vi "gantry path main.vi"() -> ()   [LabVIEW 2016]
uses:
  Classes/Controller/Motion/A3200 Folder/A3200.lvclass
  D:/Gantry_General/Classes/Controller/Motion/Motion Folder/Motion.lvclass
  Classes/Controller/Dispenser/Ultimus V2 Folder/Ultimus V2.lvclass
  Classes/Controller/I-O/NI-DAQ Folder/NI-DAQ.lvclass
  Classes/Controller/Motion/Motion Folder/Motion.lvclass
  Classes/Controller/I-O/I-O Folder/I-O.lvclass
  Classes/Controller/Dispenser/Dispenser Folder/Dispenser.lvclass
  <vilib>/Utility/file.llb/Read Delimited Spreadsheet (DBL).vi
  <vilib>/Utility/file.llb/Write Delimited Spreadsheet (DBL).vi
panel:
  out "run XYZTheta Out":dbl[](array[numeric])
  in  "string":string
  out "new path":path=path "D:/Gantry_General/Main/ms_kao/gantry path/path data/20211104-170200.046.txt"
  out "array w/ subset deleted":dbl[](array[numeric])=[1038.895, 600.353]
  out "deleted portion":dbl[](array[numeric])=[51.418, -0.0]
  out "subarray":dbl[](array[numeric])=[-0.016895, 380.054641, 0.0, -0.0]
  out "all rows":dbl[][](array[numeric])=[[1e-06, -9e-06, 0.0, 0.0], [380.023807, -5.6e-05, 1e-06, -0.0], [380.005908, 380.030345, 0.0, 1e-06], [-0.016895, 380.054641, 0.0, -0.0]]
  out "size(s)":i32[](array[numeric])=[4, 4]
  in  "cul data":bool
  in  "Tab Control":enum32{"controller", "path", "motion"}(tab)=enum."motion"
  in  "controller":T1
  in  "save data off/on":bool=TRUE
  in  "test / run 2":bool
  out "run":bool
  out "XYZU":dbl[](array[numeric])=[388.99999394968614, 389.00001276830227, 35.37117897777896, -9.350854999021411e-05]
  in  "joystick":bool
  out "Axis 2":dbl[](array[numeric])=[388.99999394968614, 389.00001276830227, 35.37117897777896, -9.350854999021411e-05]
  in  "get Axis":bool
  in  "get origin":bool
  in  "test / run":bool=TRUE
  in  "joystick off/on":bool=TRUE
  in  "XY / XYZXU":bool
  in  "Read old path":path=path "D:/Gantry_General/Main/ms_kao/gantry path/path data/20220615/calibration meterial20220111_.txt"
  in  "go path":bool
  in  "milliseconds to wait":u32=500
  out "Origin":dbl[](array[numeric])=[388.999994, 389.000013, 35.371179, -9.4e-05]
  out "file or folder exists?":bool=TRUE
  in  "add new path":bool
  in  "XY go2":bool
  in  "XYZU Position":dbl[](array[numeric])=[500.0, 500.0, 0.0]
  in  "Z Speed":dbl=40.0
  in  "XY go1":bool
  in  "XYZU go":bool
  in  "Z go":bool
  in  "XY Speed":dbl=100.0
  in  "Z Position":dbl format="%#_13g"
  in  "XY Position 1":dbl[](array[numeric])=[687.973, 195.062]
  in  "XY Position 2":dbl[](array[numeric])=[687.973, 252.062]
  in  "stop":bool
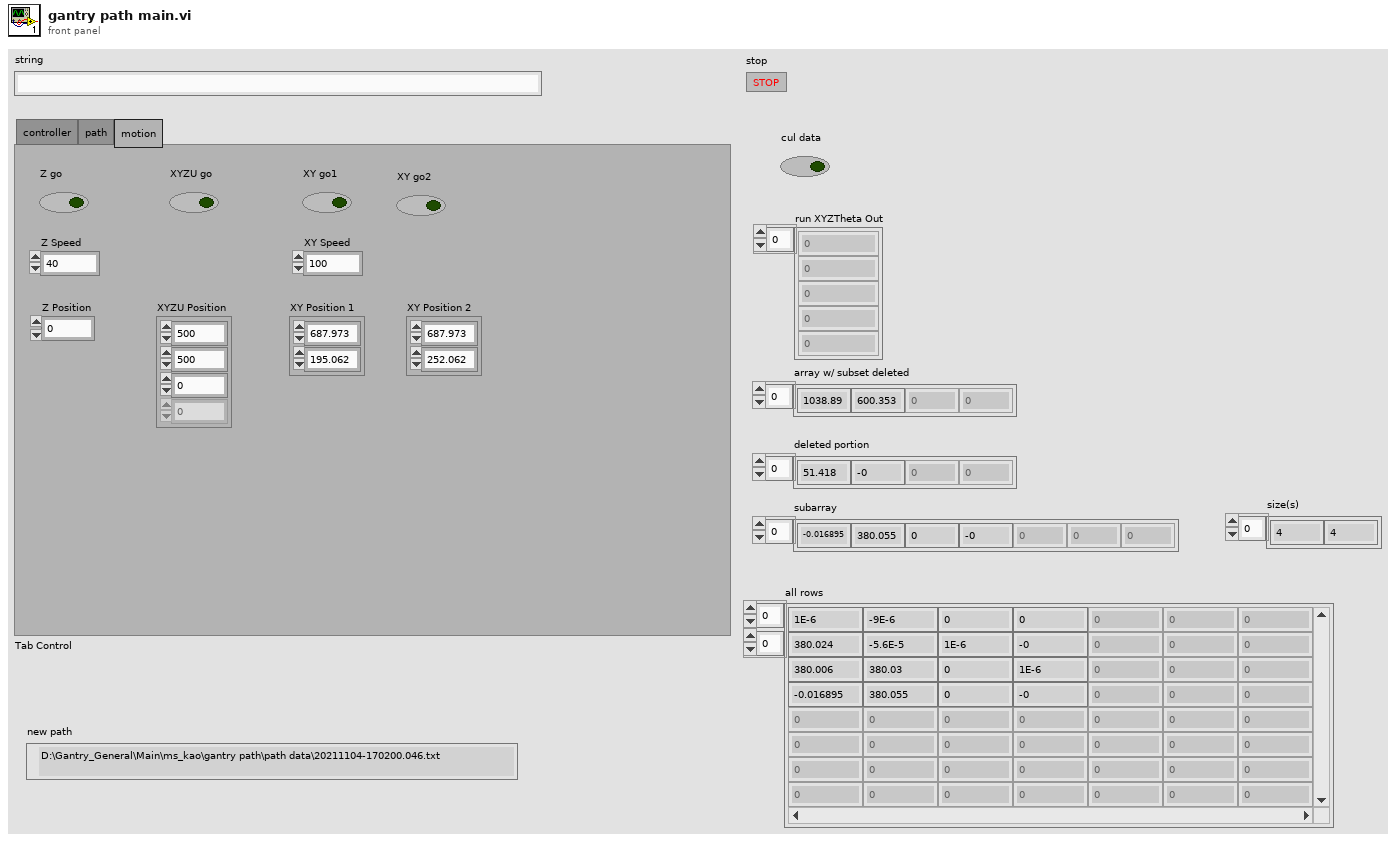
[diagram p1: front panel]
types:
  T1 = cluster{"A3200.lvclass":refnum<class "A3200.lvclass">, "Ultimus V2.lvclass":refnum<class "Ultimus V2.lvclass">, "NI-DAQ.lvclass":refnum<class "NI-DAQ.lvclass">, "Motion.lvclass":refnum<class "Motion.lvclass">, "I-O.lvclass":refnum<class "I-O.lvclass">, "Dispenser.lvclass":refnum<class "Dispenser.lvclass">}
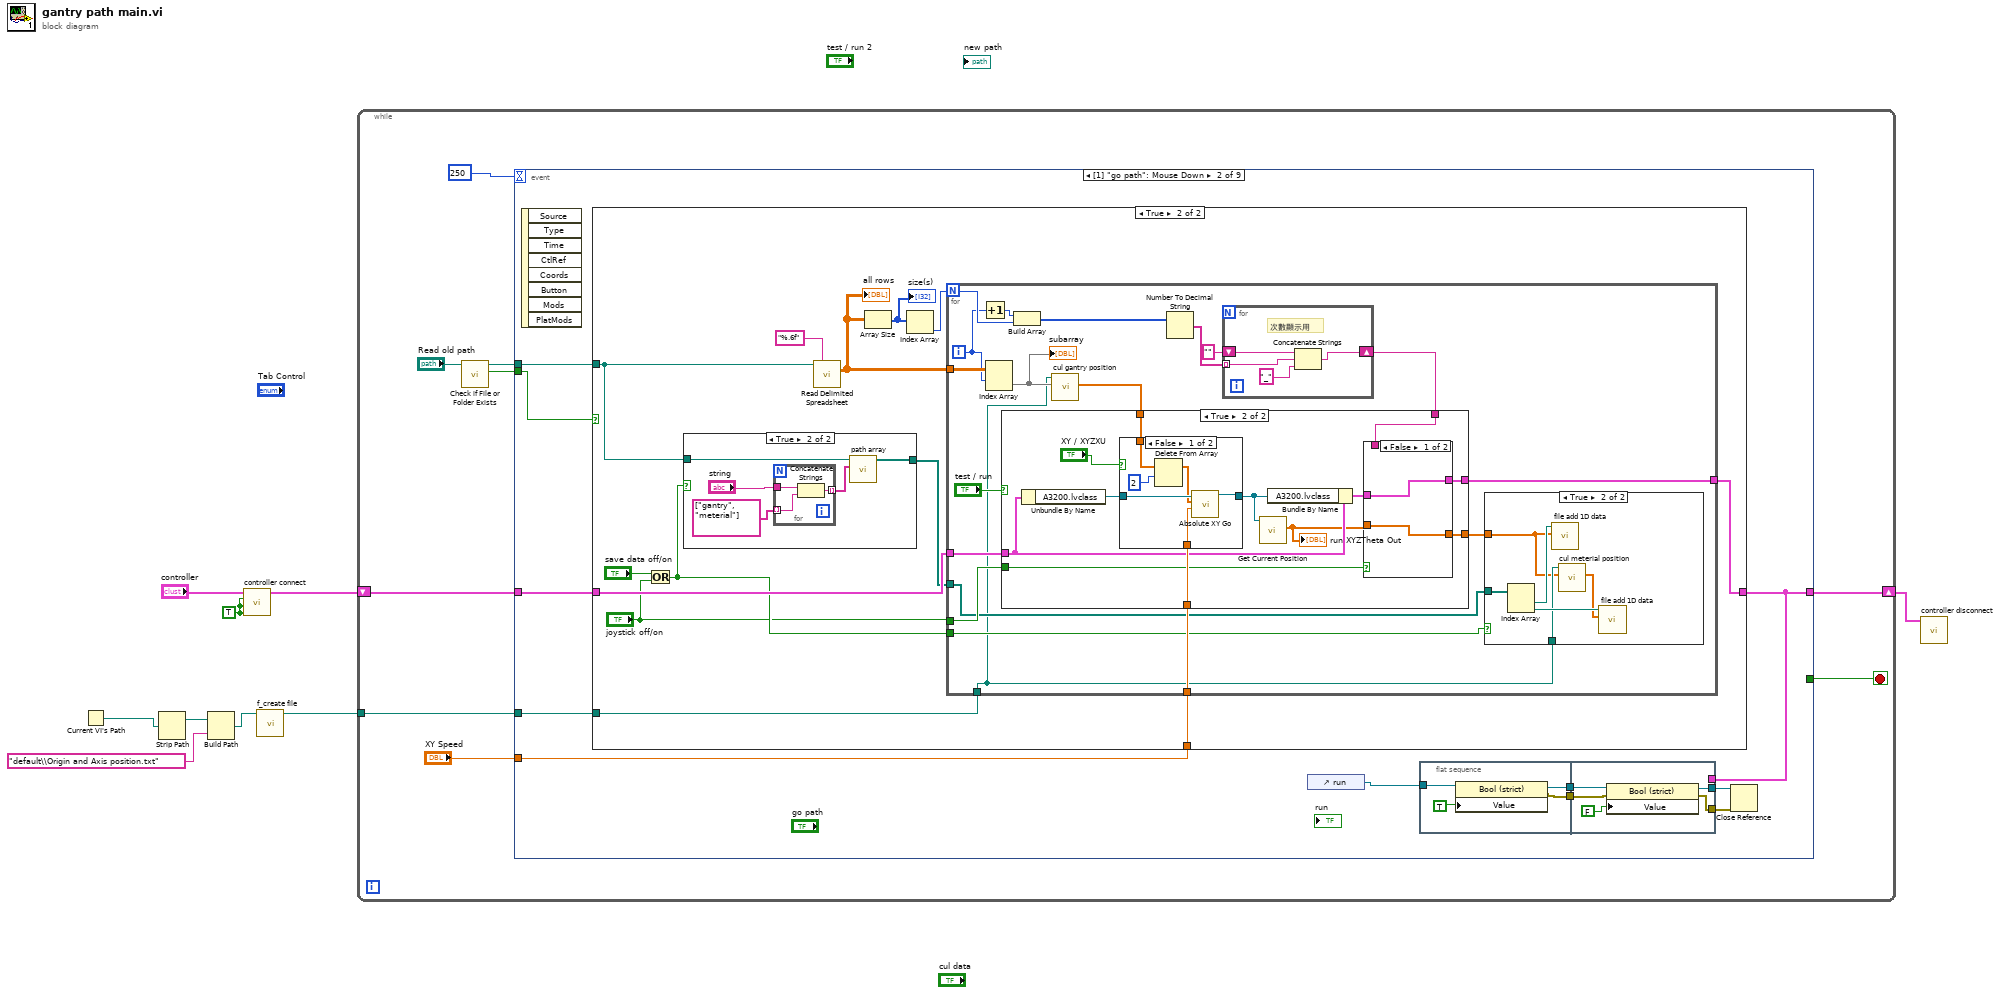
[diagram p0: block diagram]
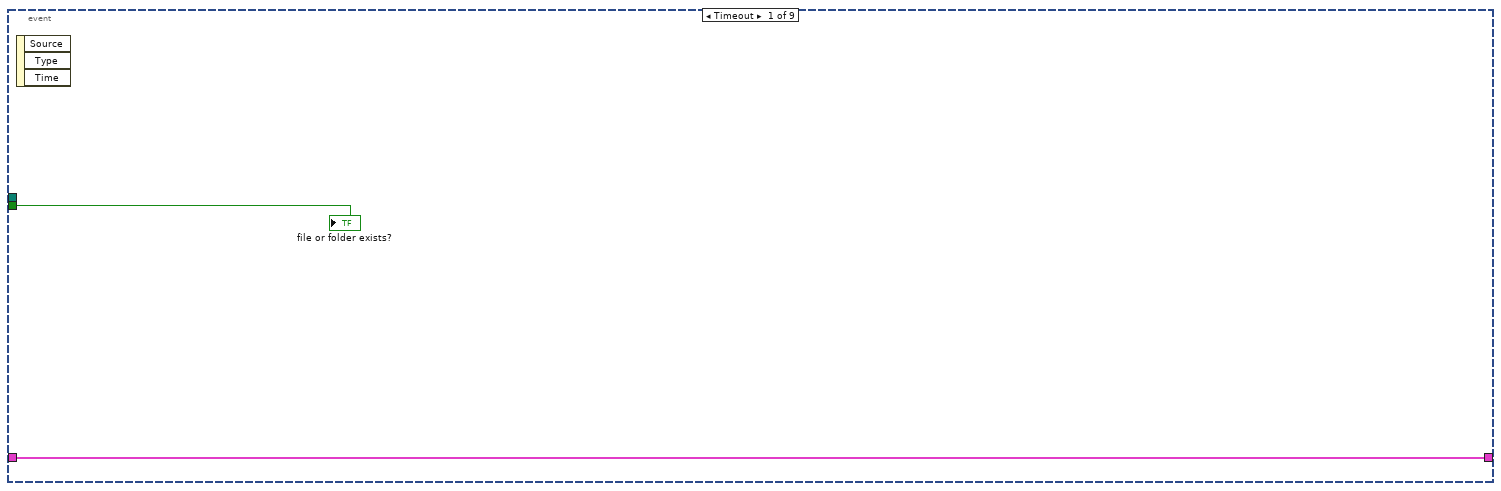
[diagram p2: hidden frame]
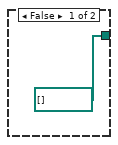
[diagram p4: hidden frame]
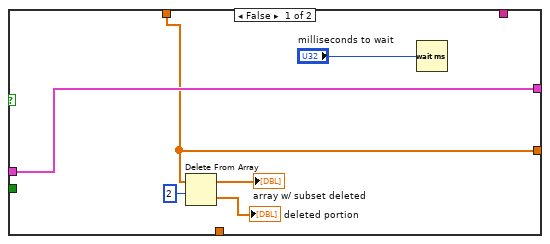
[diagram p6: hidden frame]
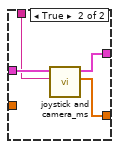
[diagram p7: hidden frame]
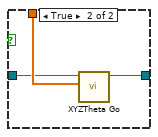
[diagram p8: hidden frame]
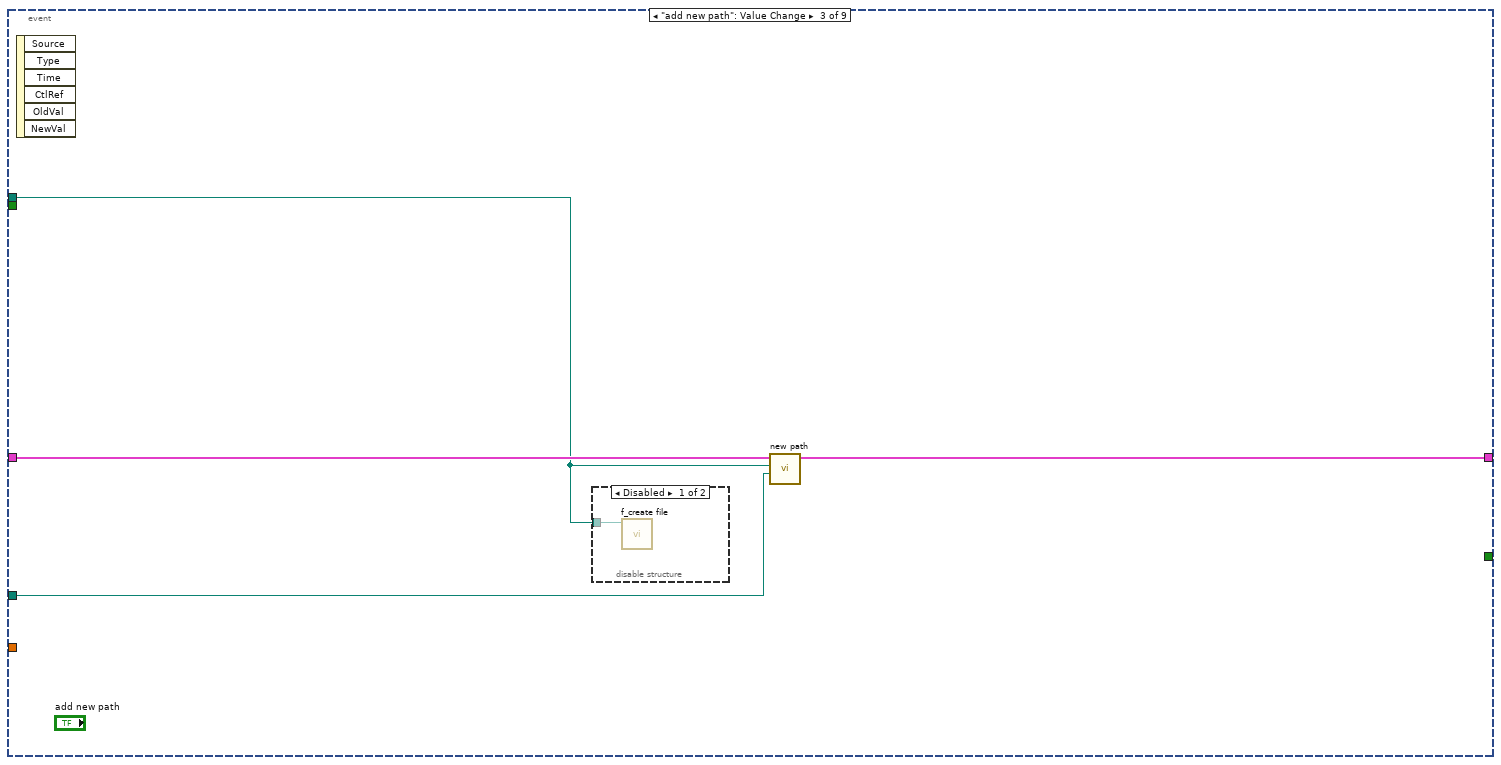
[diagram p9: hidden frame]
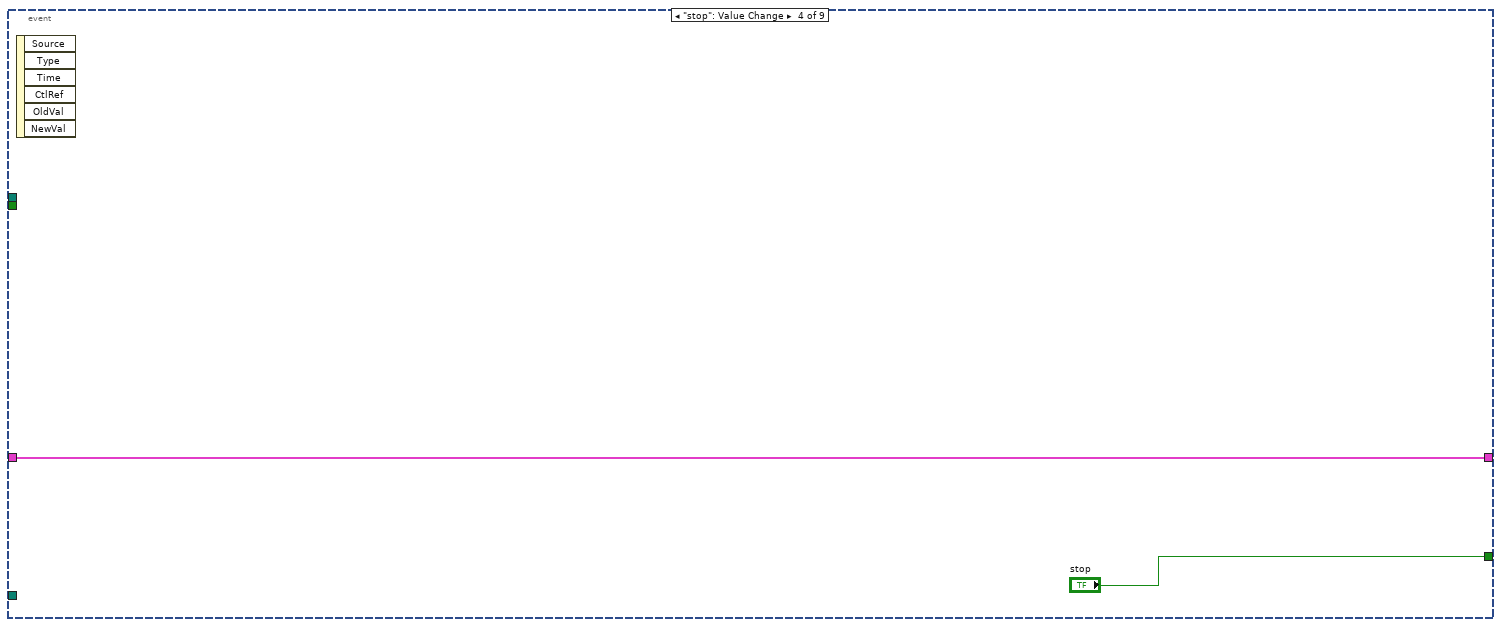
[diagram p11: hidden frame]
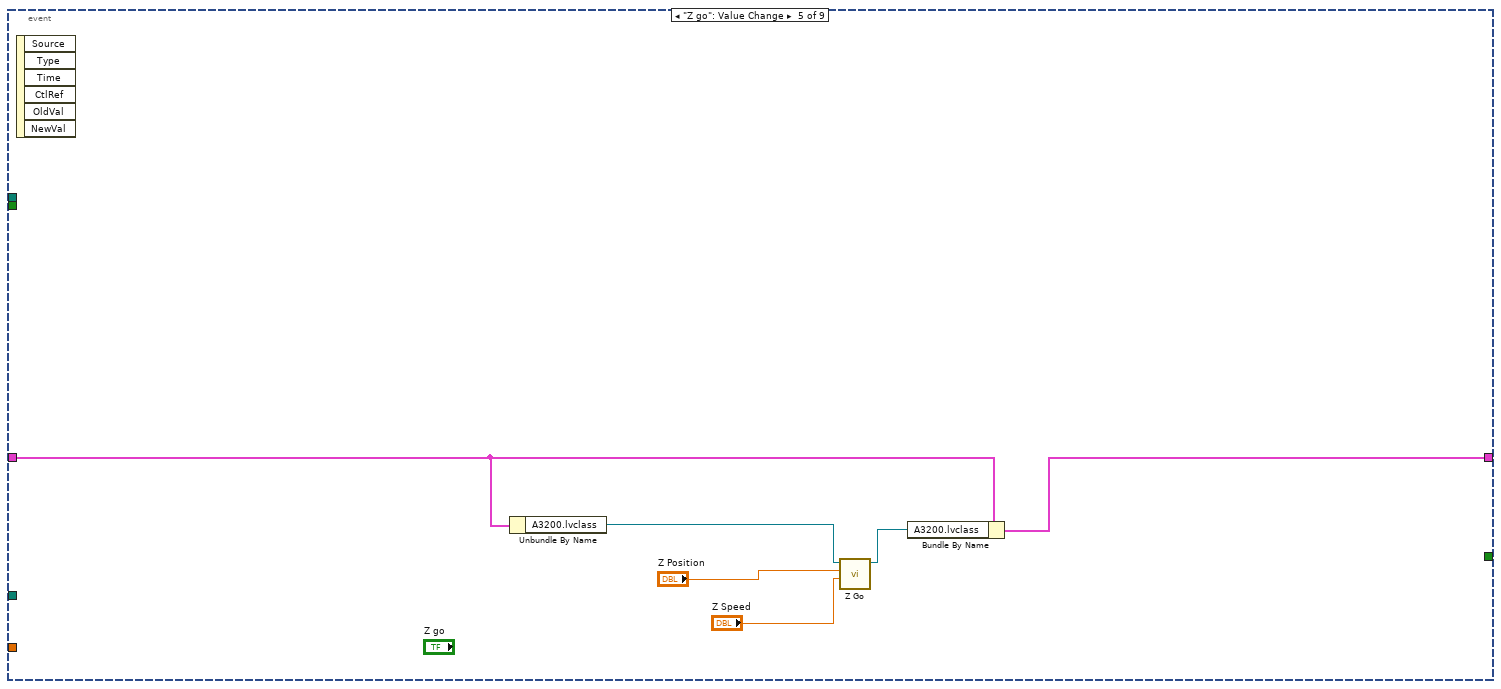
[diagram p12: hidden frame]
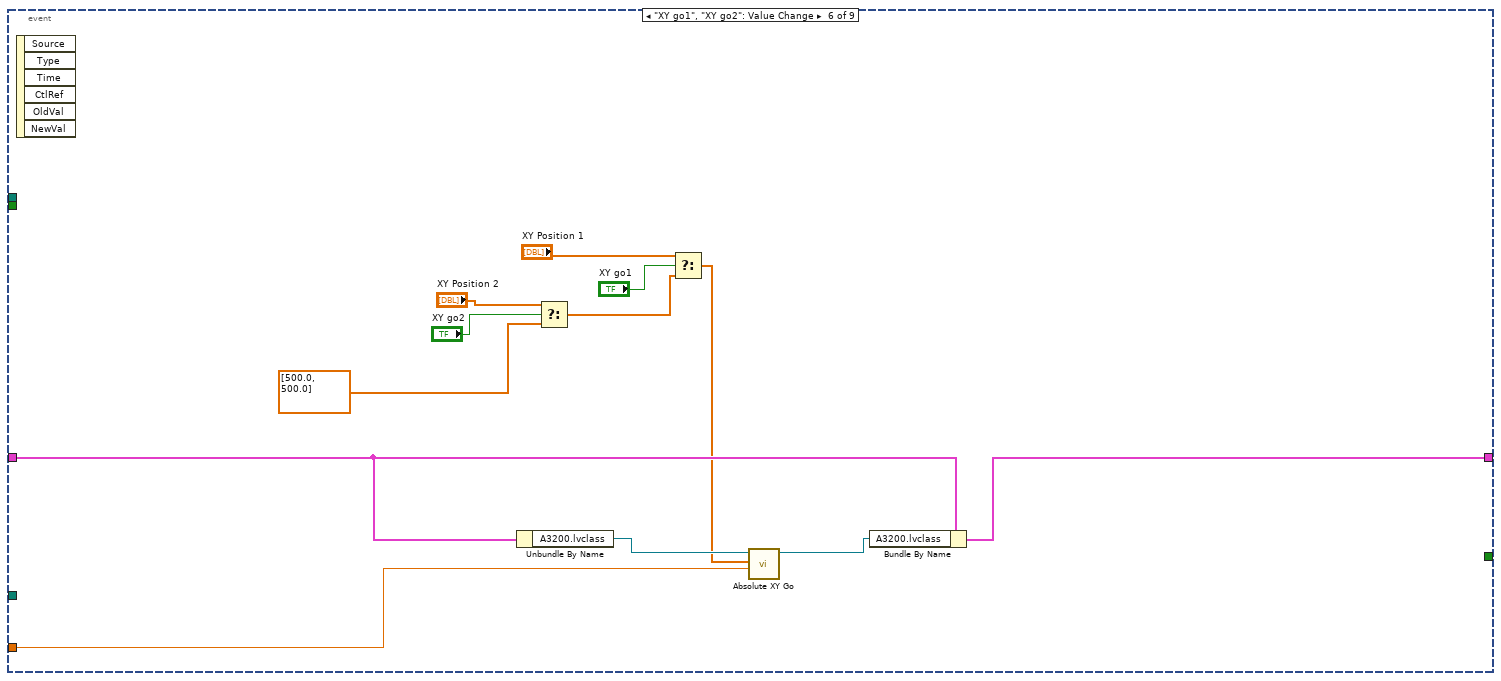
[diagram p13: hidden frame]
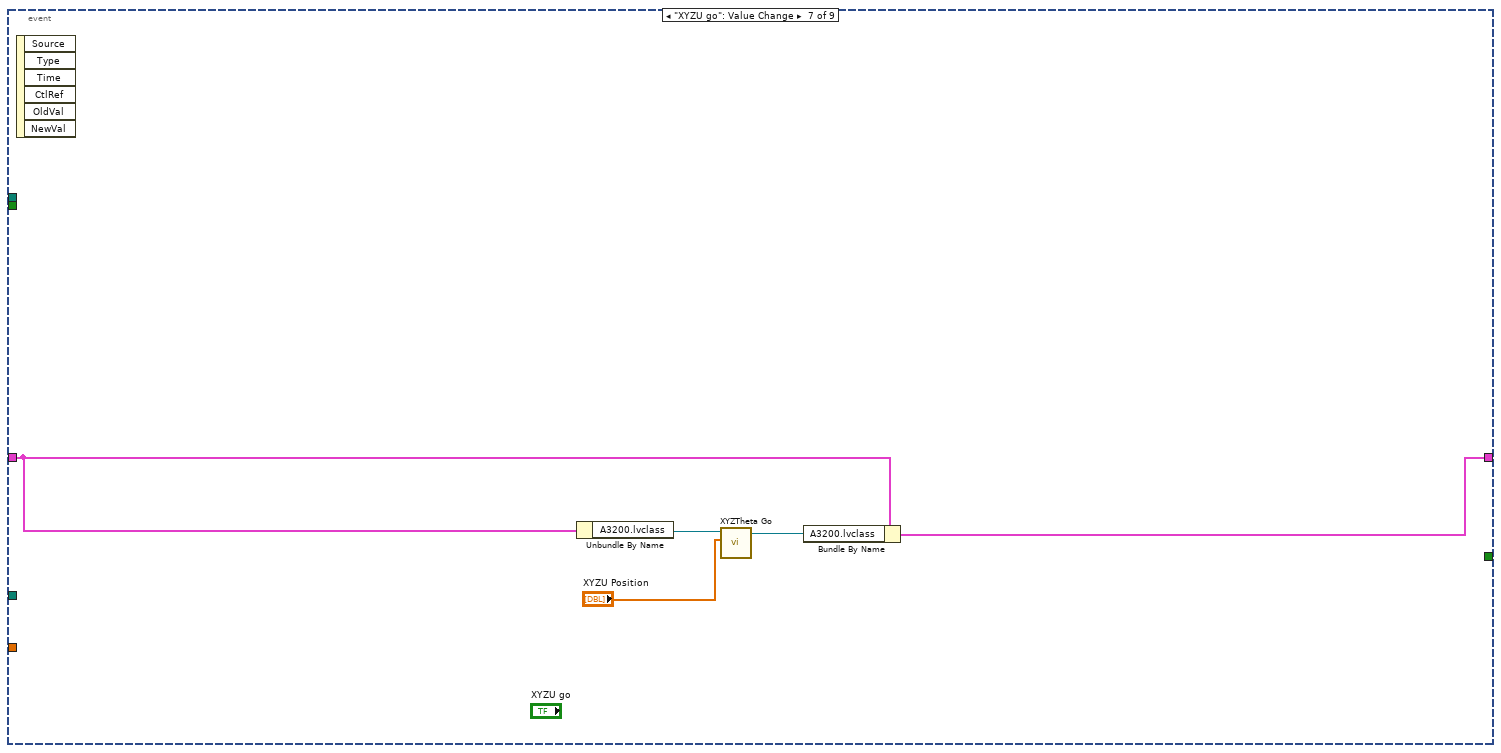
[diagram p14: hidden frame]
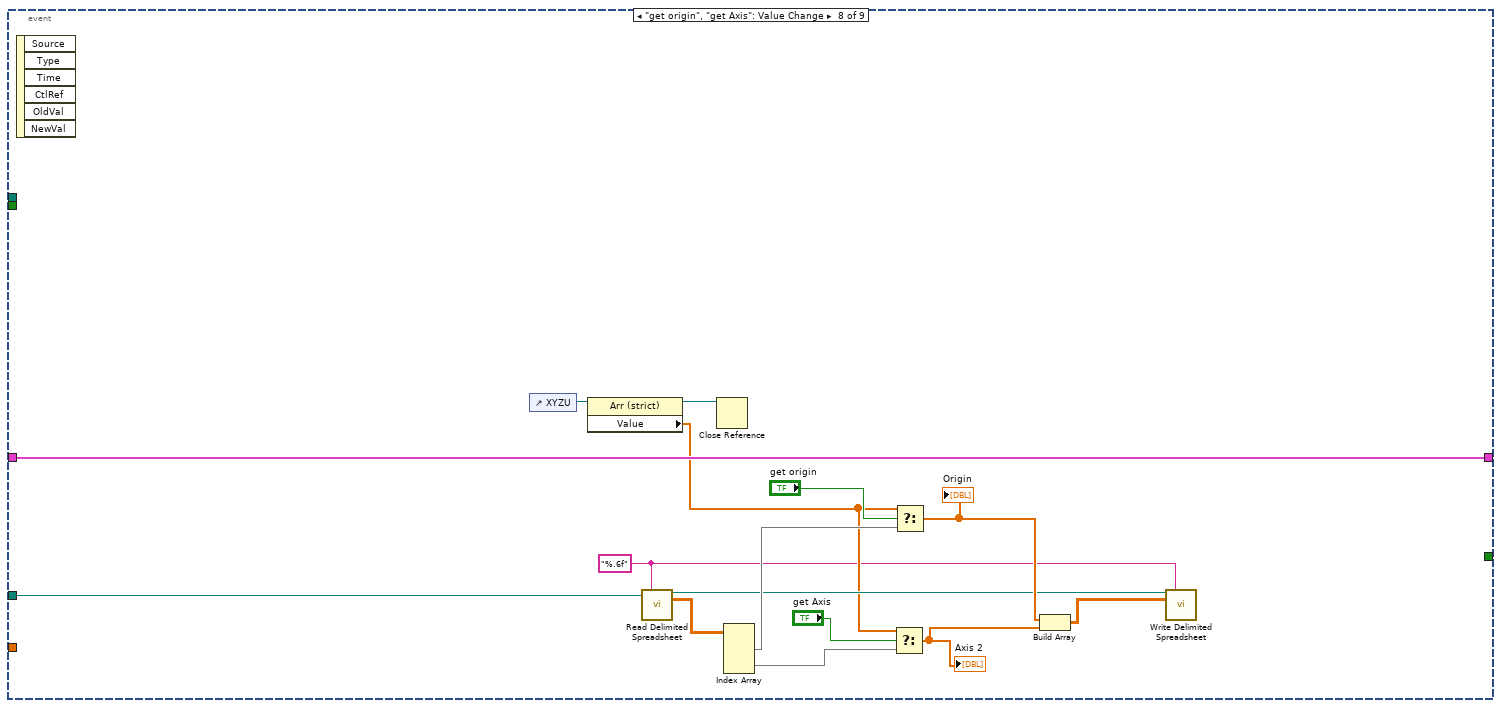
[diagram p15: hidden frame]
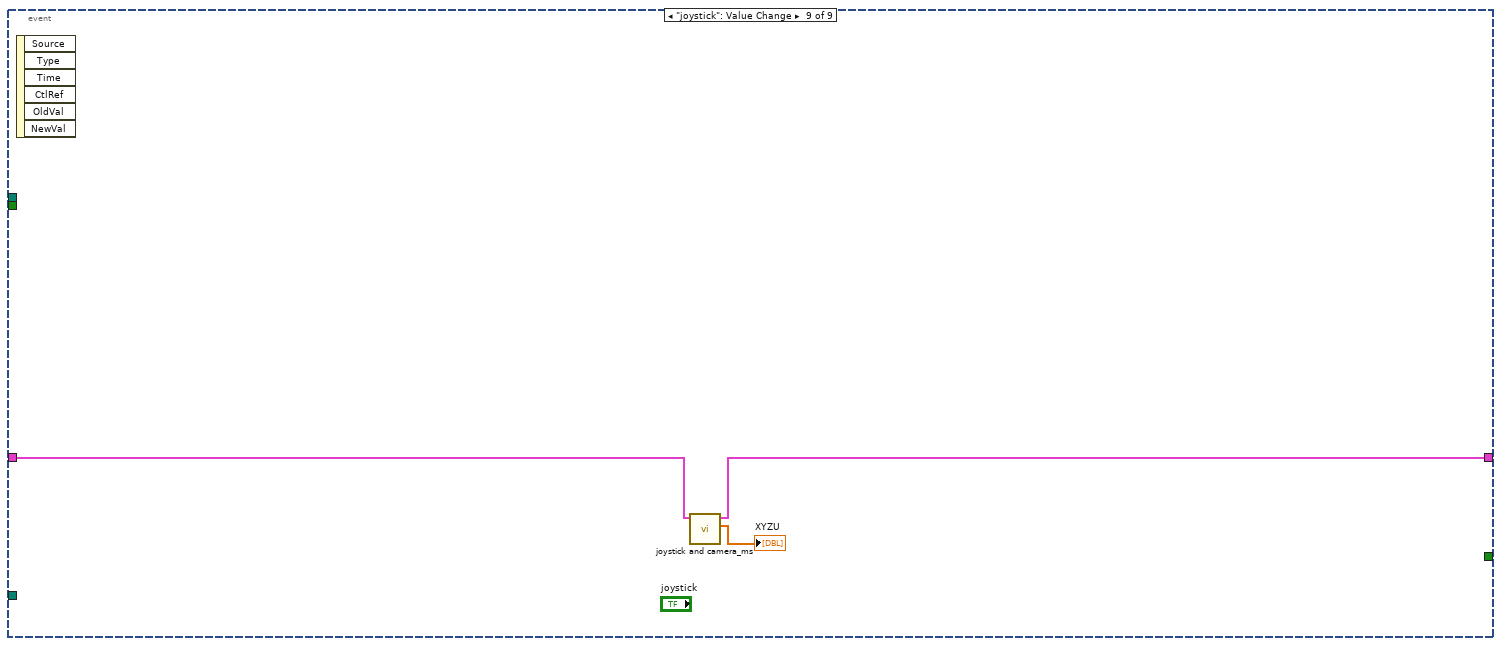
[diagram p16: hidden frame]
diagram:
  w7 = TRUE ("IO on")
  n1 = Current VI's Path() -> (path=w3:path)
  n2 = Strip Path(path=w3) -> (stripped path=w4:path)  [unwired: 1 out]
  n3 = Build Path(base path=w4, name or relative path="default\\Origin and Axis position.txt") -> (appended path=w5:path)
  n4 = call "controller connect.vi"("IO on"=w7, "dispencer on"=w7, "motion on"=w7, "controller in"="controller") -> ("controller out"=w9:T1)  [unwired: 7 in]
  n5 = call "f_create file.vi"("path"=w5) -> ("dup path"=w1:path)  [unwired: 10 in]
  n6 = while {
    shift-right: [w15] -> w6
    shift-left: w9 -> [w16]
    tunnel: w1 -> [w10]
    stop <- w18 stop-if-true
    n7 = call <vilib>:"Check if File or Folder Exists.vi"("path"="Read old path") -> ("file or folder exists?"=w12:bool, "dup path"=w11:path)  [unwired: 8 in, 1 out]
    n8 = event shown="[1] \"go path\": Mouse Down" {
      selector: _ -> [_ _ _ _ _ _ _ _ _]
      dyn-events: _ -> [_ _ _ _ _ _ _ _ _]
      timeout: 250 -> [_ _ _ _ _ _ _ _ _]
      tunnel: [_ _ _ "stop" _ _ _ _ _] -> w18
      tunnel: w11 -> [_ w28 w127 _ _ _ _ _ _]
      tunnel: w16 -> [w20 w31 w128 w131 w136 w149 w152 w160 w173]
      tunnel: [w20 w26 w129 w131 w135 w148 w155 w160 w172] -> w15
      tunnel: "XY Speed" -> [_ w30 _ _ _ w146 _ _ _]
      tunnel: w12 -> [w19 w29 _ _ _ _ _ _ _]
      tunnel: w10 -> [_ w27 w126 _ _ _ _ w162 _]
      event Timeout {
        n9 = event-data() -> ()  [unwired: 1 in, 3 out]
        "file or folder exists?" <- w19
      }
      event "go path": Mouse Down {
        n10 = event-data() -> ()  [unwired: 1 in, 8 out]
        n11 = case shown="True" w29 {
          tunnel: w28 -> [_ w46]
          tunnel: w31 -> [w41 w50]
          tunnel: [w41 w51] -> w26
          tunnel: w30 -> [_ w49]
          tunnel: w27 -> [_ w48]
          frame False {
          }
          frame True {
            n12 = Or(x="save data off/on", y="joystick off/on") -> (x .or. y?=w44:bool)
            n13 = case shown="True" w44 {
              tunnel: [path[] [] ("path array") w60] -> w47
              tunnel: w46 -> [_ w59]
              frame False {
              }
              frame True {
                n14 = for {
                  tunnel: string[] ["gantry", "meterial"] ("Array") -> [w63] mode=indexing
                  tunnel: [w62] -> w57 mode=indexing
                  tunnel: "string" -> [w61]
                  n15 = Concatenate Strings(w61, w63) -> (w62:string)
                }
                n16 = call "path array.vi"("Array"=w57, "file path (dialog if empty)"=w59) -> ("path array"=w60:path[])  [unwired: 9 in]
              }
            }
            n17 = call-poly <vilib>:"Read Delimited Spreadsheet.vi"("file path (dialog if empty)"=w46, "format (%.3f)"="%.6f") -> ("all rows"=w53:dbl[][])  [unwired: 8 in, 5 out]
            "all rows" <- w53
            n18 = Array Size(array=w53) -> (size(s)=w54:i32[])
            "size(s)" <- w54
            n19 = Index Array(array=w54) -> (element=w52:i32)  [unwired: 1 in]
            n20 = for {
              N: w52 -> [w75]
              tunnel: w53 -> [w82]
              tunnel: [w81] -> w51
              tunnel: w50 -> [w80]
              tunnel: w49 -> [w79]
              tunnel: w47 -> [w65]
              tunnel: w48 -> [w64]
              tunnel: w44 -> [w66]
              tunnel: "joystick off/on" -> [w68]
              i -> [w69]
              n21 = Increment(x=w69) -> (x+1=w70:i32)
              n22 = Index Array(array=w82, index (row)=w69) -> (element=w76:dbl[])  [unwired: 1 in]
              "subarray" <- w76
              n23 = Build Array(w70, w75) -> (w74:i32[])
              n24 = call "cul gantry position.vi"("position in"=w76, "Origin and Axis path"=w64) -> ("position out"=w77:dbl[])  [unwired: 9 in]
              n25 = Number To Decimal String(number=w74) -> (decimal integer string=w73:string[])  [unwired: 1 in]
              n26 = for {
                tunnel: w73 -> [w90] mode=indexing
                shift-right: [w92] -> w71
                shift-left: "" -> [w91]
                # "次數顯示用"
                n27 = Concatenate Strings(w91, w90, "_" ("string")) -> (w92:string)
              }
              n28 = case shown="True" "test / run" {
                tunnel: [w98 w101] -> w81
                tunnel: w80 -> [w98 w106]
                tunnel: w77 -> [w93 w109]
                tunnel: w79 -> [_ w108]
                tunnel: w71 -> [_ w103]
                tunnel: w68 -> [_ w100]
                tunnel: [w93 w99] -> w67
                frame False {
                  n29 = Delete From Array(array=w93, length=2) -> (deleted portion=→"deleted portion":dbl[], array with subset deleted=→"array w/ subset deleted":dbl[])  [unwired: 1 in]
                  n30 = Wait (ms)(milliseconds to wait="milliseconds to wait") -> ()  [unwired: 1 out]
                }
                frame True {
                  n31 = Unbundle By Name(w106) -> ("A3200.lvclass"=w107:refnum<class "A3200.lvclass">)
                  n32 = case shown="False" "XY / XYZXU" {
                    tunnel: w107 -> [w120 w124]
                    tunnel: [w119 w123] -> w105
                    tunnel: w109 -> [w121 w125]
                    tunnel: w108 -> [w118 _]
                    frame False {
                      n33 = Delete From Array(array=w121, length=2) -> (array with subset deleted=w117:dbl[])  [unwired: 1 in, 1 out]
                      n34 = call-dynamic "Absolute XY Go.vi"("Speed"=w118, "XY"=w117, "Gantry in"=w120) -> ("Gantry out"=w119:refnum<class "A3200.lvclass">)  [unwired: 7 in, 1 out]
                    }
                    frame True {
                      n35 = call "XYZTheta Go.vi"("XYZTheta In"=w125, "Motion in"=w124) -> ("Motion out"=w123:refnum<class "A3200.lvclass">)  [unwired: 7 in, 2 out]
                    }
                  }
                  n36 = call-dynamic "Get Current Position.vi"("Gantry in"=w105) -> ("XYZTheta Out"=w104:dbl[])  [unwired: 8 in, 2 out]
                  "run XYZTheta Out" <- w104
                  n37 = Bundle By Name(cluster=w106, "A3200.lvclass"=w105) -> (w102:T1)
                  n38 = case shown="False" w100 {
                    tunnel: [w112 w116] -> w101
                    tunnel: w102 -> [w112 w115]
                    tunnel: [w111 w114] -> w99
                    tunnel: w103 -> [_ w113]
                    tunnel: w104 -> [w111 _]
                    frame False {
                    }
                    frame True {
                      n39 = call "joystick and camera_ms.vi"("Text"=w113, "controller in"=w115) -> ("Gantry"=w114:dbl[], "controller out"=w116:T1)  [unwired: 8 in]
                    }
                  }
                }
              }
              n40 = case shown="True" w66 {
                tunnel: w65 -> [_ w84]
                tunnel: w64 -> [_ w85]
                tunnel: w67 -> [_ w83]
                frame False {
                }
                frame True {
                  n41 = Index Array(array=w84) -> (element #1=w88:path, element #2=w87:path)  [unwired: 2 in]
                  n42 = call "file add 1D data.vi"("element"=w83, "file path (dialog if empty)"=w88) -> ()  [unwired: 10 in]
                  n43 = call "cul meterial position.vi"("position in"=w83, "Origin and Axis path"=w85) -> ("position out"=w86:dbl[])  [unwired: 9 in]
                  n44 = call "file add 1D data.vi"("element"=w86, "file path (dialog if empty)"=w87) -> ()  [unwired: 10 in]
                }
              }
            }
          }
        }
        n45 = control-ref of="run"() -> (w25:refnum<vi>)
        n46 = flat-sequence {
          tunnel: w25 -> [w34]
          tunnel: [w33] -> w24
          tunnel: [w32] -> w23
          tunnel: w26 -> [_]
          tunnel: w24 -> [w40]
          tunnel: w23 -> [w39]
          tunnel: [w37] -> w22
          tunnel: [w36] -> w21
          frame #0 {
            n47 = property class="Bool (strict)"(reference=w34, "Value"=TRUE ("run")) -> (reference out=w33:refnum<vi>, error out=w32:errorcluster)  [unwired: 1 in]
          }
          frame #1 {
            n48 = property class="Bool (strict)"(reference=w40, error in=w39, "Value"=FALSE ("run")) -> (reference out=w37:refnum<vi>, error out=w36:errorcluster)
          }
        }
        n49 = Close Reference(reference=w22, error in (no error)=w21) -> ()  [unwired: 1 out]
      }
      event "add new path": Value Change {
        n50 = event-data() -> ()  [unwired: 1 in, 6 out]
        n51 = disable-structure shown="Disabled" {
          disable-tunnel: w127 -> [w130 _]
          frame Disabled {
            n52 = call "f_create file.vi"("path"=w130) -> ()  [unwired: 10 in, 1 out]
          }
          frame Enabled {
          }
        }
        n53 = call "new path.vi"("Origin and Axis path"=w126, "position path"=w127, "controller"=w128) -> ("controller 2"=w129:T1)  [unwired: 8 in]
      }
      event "stop": Value Change {
        n54 = event-data() -> ()  [unwired: 1 in, 6 out]
      }
      event "Z go": Value Change {
        n55 = event-data() -> ()  [unwired: 1 in, 6 out]
        n56 = Unbundle By Name(w136) -> ("A3200.lvclass"=w138:refnum<class "A3200.lvclass">)
        n57 = call-dynamic "Z Go.vi"("Speed"="Z Speed", "Position"="Z Position", "Gantry in"=w138) -> ("Gantry out"=w137:refnum<class "A3200.lvclass">)  [unwired: 7 in, 1 out]
        n58 = Bundle By Name(cluster=w136, "A3200.lvclass"=w137) -> (w135:T1)
      }
      event "XY go1", "XY go2": Value Change {
        n59 = event-data() -> ()  [unwired: 1 in, 6 out]
        n60 = Unbundle By Name(w149) -> ("A3200.lvclass"=w150:refnum<class "A3200.lvclass">)
        n61 = Select(t="XY Position 2", s="XY go2", f=dbl[] [500.0, 500.0]) -> (s? t:f=w141:dbl[])
        n62 = Select(t="XY Position 1", s="XY go1", f=w141) -> (s? t:f=w145:dbl[])
        n63 = call-dynamic "Absolute XY Go.vi"("Speed"=w146, "XY"=w145, "Gantry in"=w150) -> ("Gantry out"=w147:refnum<class "A3200.lvclass">)  [unwired: 7 in, 1 out]
        n64 = Bundle By Name(cluster=w149, "A3200.lvclass"=w147) -> (w148:T1)
      }
      event "XYZU go": Value Change {
        n65 = event-data() -> ()  [unwired: 1 in, 6 out]
        n66 = Unbundle By Name(w152) -> ("A3200.lvclass"=w153:refnum<class "A3200.lvclass">)
        n67 = call "XYZTheta Go.vi"("XYZTheta In"="XYZU Position", "Motion in"=w153) -> ("Motion out"=w154:refnum<class "A3200.lvclass">)  [unwired: 7 in, 2 out]
        n68 = Bundle By Name(cluster=w152, "A3200.lvclass"=w154) -> (w155:T1)
      }
      event "get origin", "get Axis": Value Change {
        w156 = "%.6f" ("format (%.3f)")
        n69 = event-data() -> ()  [unwired: 1 in, 6 out]
        n70 = control-ref of="XYZU"() -> (w159:refnum<vi>)
        n71 = property class="Arr (strict)"(reference=w159) -> (reference out=w158:refnum<vi>, "Value"=w157:dbl[])  [unwired: 1 in, 1 out]
        n72 = call-poly <vilib>:"Read Delimited Spreadsheet.vi"("file path (dialog if empty)"=w162, "format (%.3f)"=w156) -> ("new file path (Not A Path if cancelled)"=w161:path, "all rows"=w165:dbl[][])  [unwired: 8 in, 4 out]
        n73 = Close Reference(reference=w158) -> ()  [unwired: 1 in, 1 out]
        n74 = Index Array(array=w165) -> (element #1=w164:dbl[], element #2=w163:dbl[])  [unwired: 4 in]
        n75 = Select(t=w157, s="get Axis", f=w163) -> (s? t:f=w167:dbl[])
        "Axis 2" <- w167
        n76 = Select(t=w157, s="get origin", f=w164) -> (s? t:f=w168:dbl[])
        "Origin" <- w168
        n77 = Build Array(w168, w167) -> (w166:dbl[][])
        n78 = call-poly <vilib>:"Write Delimited Spreadsheet.vi"("file path (dialog if empty)"=w161, "format (%.3f)"=w156, "2D data"=w166) -> ()  [unwired: 11 in, 2 out]
      }
      event "joystick": Value Change {
        n79 = event-data() -> ()  [unwired: 1 in, 6 out]
        n80 = call "joystick and camera_ms.vi"("controller in"=w173) -> ("Gantry"=→"XYZU":dbl[], "controller out"=w172:T1)  [unwired: 9 in]
      }
    }
  }
  n81 = call "controller disconnect.vi"("controller 2"=w6) -> ()  [unwired: 11 in]
